vi "PowerMeter_Measurement.vi"() -> ()   [LabVIEW 2017]
panel:
  out "Power Value":dbl caption="Optical Power [W]" format="%#_4p"
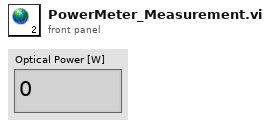
[diagram p1: front panel]
diagram:
